vi "OAT Extract Order Waveforms (Combined Orders).vi"(0 "scaled signal [EU]":waveform(dbl)={"t0"=timestamp(0 s since 1904-01-01), "dt"=0.0, "Y"=[]}, 5 "speed profile":T3 {"speed [RPM]" format="%.2f"; "time [s]" format="%.2f"}, 9 "orders to extract":cluster{"combined orders":dbl[]}[](array[cluster]), 11 "error in (no error)":errorcluster, 12 "bandwidth":T2={"bandwidth value"=0.5, "bandwidth unit"=enum."Order"} {"bandwidth value" min=0.0 format="%.2f"}, 13 "window info":T1={"window type"=10, "window length"=2048} {"window type" items=["None"=0, "Hanning"=1, "Hamming"=2, "Blackman-Harris"=3, "Exact Blackman"=4, "Blackman"=5, "Flat Top"=6, "4 Term B-Harris"=7, "7 Term B-Harris"=8, "Low Sidelobe"=9, "Gaussian"=62]; "window length" min=0}) -> (4 "order waveforms":waveform(dbl)[](array[waveform]), 6 "order list":string[](array[string]), 10 "unit label":string, 14 "actual window info":T1={"window type"=10, "window length"=2048} {"window type" items=["None"=0, "Hanning"=1, "Hamming"=2, "Blackman-Harris"=3, "Exact Blackman"=4, "Blackman"=5, "Flat Top"=6, "4 Term B-Harris"=7, "7 Term B-Harris"=8, "Low Sidelobe"=9, "Gaussian"=62]; "window length" min=0}, 15 "error out":errorcluster)   [LabVIEW 2017, in "SoundVib_Gabor.lvlib"]
doc: "Extracts order waveforms from specified orders in the <B>scaled signal [EU]</B>. This VI can return order waveforms of a single order or combined orders. Use <B>orders to extract</B> to specify the desired orders. This VI does not maintain state internally; you can use this VI in a loop to process multiple blocks. Wire data to the <B>scaled signal [EU]</B> input to determine the polymorphic instance to use or manually select the instance."
uses:
  <vilib>/addons/Sound and Vibration/Order Analysis/Gabor Order Tracking/SoundVib_Gabor.lvlib
  <vilib>/addons/Sound and Vibration/Order Analysis/Tach Process/SubVIs/speed profile.ctl
  <vilib>/addons/Sound and Vibration/Order Analysis/Ref Gabor Order Tracking/window information.ctl
  <vilib>/addons/Sound and Vibration/Order Analysis/Ref Gabor Order Tracking/Mask Bandwidth.ctl
  <vilib>/addons/_NISVFA/_Shared subVIs/Common/svc_Engineering Units to Unit Label.vi
  <vilib>/addons/_NISVFA/_Shared subVIs/Common/svc_Unit Label to Engineering Units.vi
  <vilib>/addons/Sound and Vibration/Order Analysis/Tach Process/SoundVib_TachProcess.lvlib
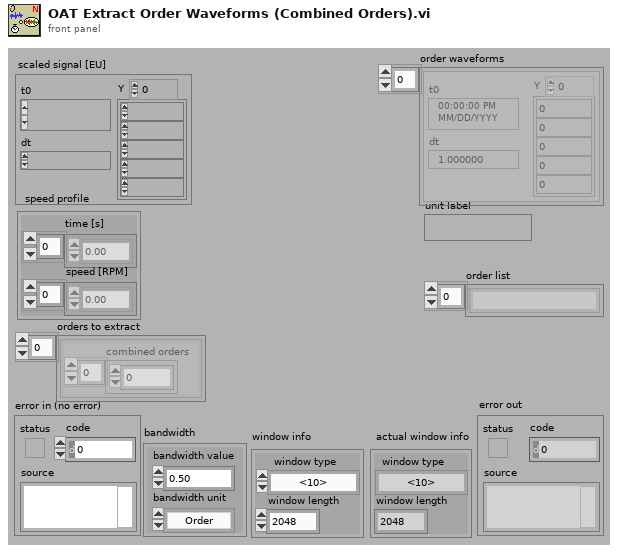
[diagram p1: front panel]
types:
  T1 = typedef "SoundVib_Gabor.lvlib/window information.ctl" = cluster{"window type":u32, "window length":i32}
  T2 = typedef "SoundVib_Gabor.lvlib/Mask Bandwidth.ctl" = cluster{"bandwidth value":dbl, "bandwidth unit":enum16{"Order", "Hz"}}
  T3 = typedef "SoundVib_TachProcess.lvlib/speed profile.ctl" = cluster{"time [s]":dbl[], "speed [RPM]":dbl[]}
  T4 = typedef "svc_Channel Info.ctl" = cluster{"sensor sensitivity":dbl, "engineering units":T5, "dB reference":dbl, "custom label":string, "weighting filter":T6, "pregain":dbl}
  T5 = typedef "svc_Engineering Units Text Ring.ctl" = u16
  T6 = typedef "svc_Weighting Filter Text Ring.ctl" = u16
  T7 = typedef "SoundVib_Gabor.lvlib/GT RefNum.ctl" = refnum<k1>
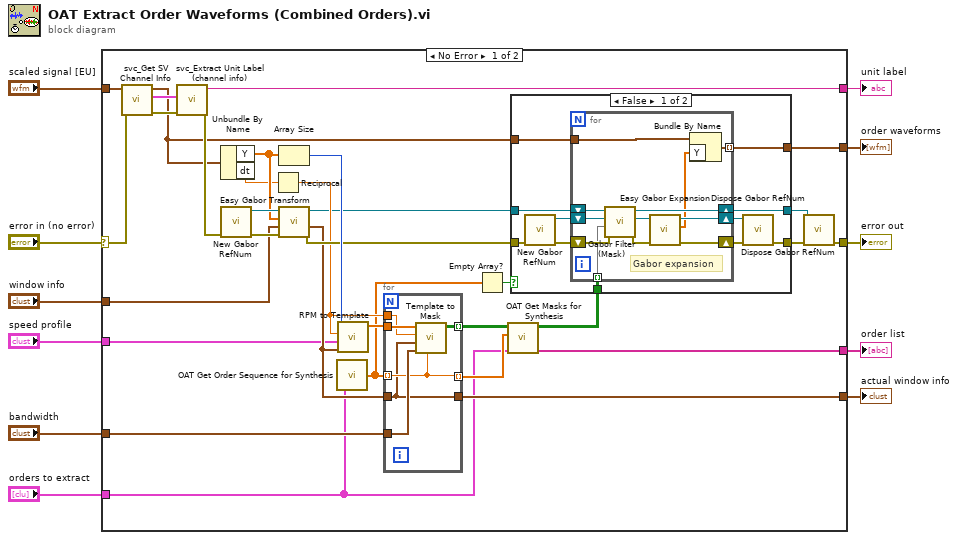
[diagram p0: block diagram]
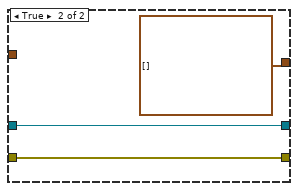
[diagram p2: hidden frame]
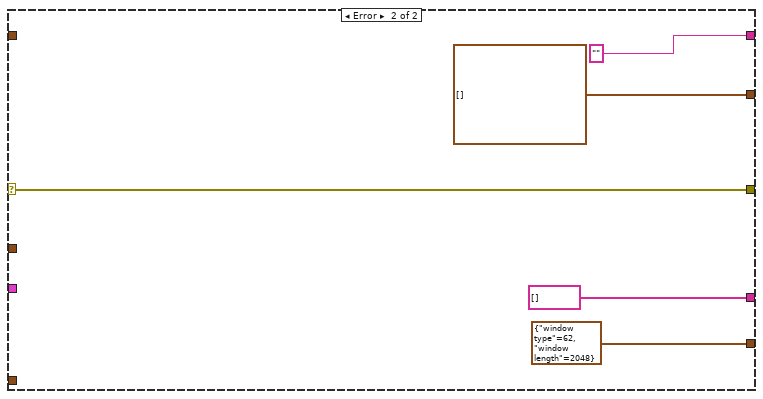
[diagram p3: hidden frame]
diagram:
  n1 = case shown="No Error" "error in (no error)" {
    selector: "error in (no error)" -> [w21 w80]
    tunnel: [w15 T1 {"window type"=62, "window length"=2048} ("actual window")] -> w11
    tunnel: "orders to extract" -> [w13 _]
    tunnel: "scaled signal [EU]" -> [w28 _]
    tunnel: "speed profile" -> [w26 _]
    tunnel: [w25 "" ("unit label")] -> w7
    tunnel: [w24 waveform(dbl)[] []] -> w6
    tunnel: [w17 string[] []] -> w5
    tunnel: "window info" -> [w23 _]
    tunnel: "bandwidth" -> [w22 _]
    tunnel: [w20 w80] -> w1
    frame No Error {
      n2 = call <vilib>:"svc_Get SV Channel Info.vi"("error in (no error)"=w21, "scaled signal [EU]"=w28) -> ("error out"=w42:errorcluster, "channel info"=w43:T4, "dup scaled signal [EU]"=w31:waveform(dbl))  [unwired: 4 in, 3 out]
      n3 = call <vilib>:"svc_Extract Unit Label (channel info).vi"("error in (no error)"=w42, "channel info"=w43) -> ("error out"=w41:errorcluster, "unit label"=w25:string)  [unwired: 7 in, 1 out]
      n4 = Unbundle By Name(w31) -> ("Y"=w39:dbl[], "dt"=w37:dbl)
      n5 = call <vilib>:"New Gabor RefNum.vi"("error in (no error)"=w41) -> ("error out"=w27:errorcluster, "RefNum"=w40:T7)  [unwired: 8 in]
      n6 = Reciprocal(x=w37) -> (1/x=w33:dbl)
      n7 = Array Size(array=w39) -> (size(s)=w38:i32)
      n8 = call <vilib>:"Easy Gabor Transform.vi"("error in (no error)"=w27, "window info"=w23, "x[n]"=w39, "RefNum in"=w40) -> ("error out"=w36:errorcluster, "actual window"=w35:T1, "RefNum out"=w32:T7)  [unwired: 3 in, 2 out]
      n9 = call <vilib>:"OAT Get Order Sequence for Synthesis.vi"("orders to extract"=w13) -> ("order sequence"=w12:dbl[])  [unwired: 4 in]
      n10 = call <vilib>:"RPM to Template.vi"("window info"=w35, "speed profile"=w26, "sampling frequency [Hz]"=w33, "signal length"=w38) -> ("Gabor template"=w34:dbl[])  [unwired: 6 in, 1 out]
      n11 = for {
        tunnel: w12 -> [w71] mode=indexing
        tunnel: w35 -> [w70]
        tunnel: w34 -> [w75]
        tunnel: w33 -> [w74]
        tunnel: w22 -> [w73]
        tunnel: [w72] -> w19 mode=indexing
        tunnel: [w71] -> w16 mode=indexing
        tunnel: [w70] -> w15
        n12 = call <vilib>:"Template to Mask.vi"("order (1.0)"=w71, "bandwidth"=w73, "window info"=w70, "sampling frequency [S/s]"=w74, "Gabor template"=w75) -> ("mask array"=w72:bool[][])  [unwired: 6 in]
      }
      n13 = Empty Array?(array=w12) -> (empty?=w14:bool)
      n14 = call <vilib>:"OAT Get Masks for Synthesis.vi"("orders to extract"=w13, "order sequence"=w16, "mask"=w19) -> ("order list"=w17:string[], "synthesis mask"=w18:bool[][][])  [unwired: 7 in]
      n15 = case shown="False" w14 {
        tunnel: w36 -> [w54 w68]
        tunnel: w32 -> [w53 w69]
        tunnel: w31 -> [w50 _]
        tunnel: [w47 w68] -> w30
        tunnel: [w46 w69] -> w29
        tunnel: [w45 waveform(dbl)[] []] -> w24
        tunnel: w18 -> [w44 _]
        frame False {
          n16 = call <vilib>:"New Gabor RefNum.vi"("error in (no error)"=w54) -> ("error out"=w51:errorcluster, "RefNum"=w52:T7)  [unwired: 8 in]
          n17 = for {
            tunnel: w44 -> [w63] mode=indexing
            shift-right: [w61] -> w48
            shift-left: w51 -> [w64]
            tunnel: w50 -> [w57]
            tunnel: [w55] -> w45 mode=indexing
            shift-right: [w59] -> w46
            shift-left: w53 -> [w66]
            shift-right: [w58] -> w49
            shift-left: w52 -> [w65]
            # "Gabor expansion"
            n18 = call <vilib>:"Gabor Filter (Mask).vi"("error in (no error)"=w64, "mask array"=w63, "dest RefNum in"=w65, "src RefNum in"=w66) -> ("error out"=w60:errorcluster, "dest RefNum out"=w62:T7, "RefNum out"=w59:T7)  [unwired: 5 in]
            n19 = call <vilib>:"Easy Gabor Expansion.vi"("error in (no error)"=w60, "RefNum in"=w62) -> ("error out"=w61:errorcluster, "time waveform"=w56:dbl[], "RefNum out"=w58:T7)  [unwired: 7 in]
            n20 = Bundle By Name(cluster=w57, "Y"=w56) -> (w55:waveform(dbl))
          }
          n21 = call <vilib>:"Dispose Gabor RefNum.vi"("error in (no error)"=w48, "RefNum in"=w49) -> ("error out"=w47:errorcluster)  [unwired: 6 in]
        }
        frame True {
        }
      }
      n22 = call <vilib>:"Dispose Gabor RefNum.vi"("error in (no error)"=w30, "RefNum in"=w29) -> ("error out"=w20:errorcluster)  [unwired: 6 in]
    }
    frame Error {
    }
  }
  "unit label" <- w7
  "order waveforms" <- w6
  "error out" <- w1
  "order list" <- w5
  "actual window info" <- w11
